vi "QCA - DUT Generate Tx Command.vi"(10 "Freq Index":i32, 11 "Standard Index":i32) -> (3 "Command Sent":string)   [LabVIEW 2011]
uses:
  niWLAN/WLAN -  niWLAN - INC - Select Measurement.ctl
panel:
  out "size(s)":i32
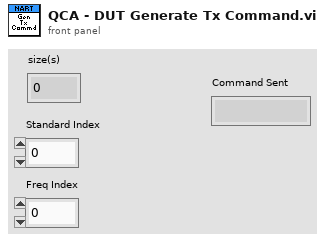
[diagram p1: front panel]
types:
  T1 = typedef "WLAN -  niWLAN - INC - Select Measurement.ctl" = cluster{"Tx_ 802.11a/g OFDM":bool, "Tx_ 802.11b DSSS/CCK":bool, "Tx_ 802.11n OFDM ":bool, "Tx_ 802.11ac OFDM ":bool}
  T2 = typedef "WLAN - TV - RW - INC - TV_DataType_Cluster.ctl" = cluster{"Standard":i32, "Channel Frequency(Hz)":dbl, "Power Level(dBm)":dbl, "Channel Bandwidth (Hz)":dbl, "Idle Interval(s)":dbl, "OFDM Data Rate (Mbps)":i32, "OFDM Payload Length (bytes)":i32, "Number of Packets":i32, "MCS Index":i32, "Guard Interval (s)":dbl, "80211n PLCP Frame Format":i32, "FEC Coding Type":i32, "DSSS Data Rate (Mbps)":i32, "DSSS Payload Length (bytes)":i32, "N_SS":i32}
  T3 = typedef "WLAN - TV - RW - INC - Tx_Measurement_Cluster.ctl" = cluster{"OFDM Advanced Controls(11ag)":T4, "DSSS Demod Parameters":T5, "OFDM Advanced Controls (11n)":T4, "OFDM Advanced Controls(11ac)":cluster{"OFDM Auto Compute Acquisition Length Enabled":i32, "OFDM Maximum Symbols Used":i32, "OFDM Time Tracking Enabled":i32, "OFDM Channel Tracking Enabled":i32, "OFDM Amplitude Tracking Enabled":i32, "OFDM CFO Estimation Method":i32, "OFDM Phase Tracking Method":i32, "OFDM Header Detection Enabled":i32, "OFDM MAC FCS Check Enabled":i32, "#Avg":i32, "#Iterations":i32}}
  T4 = typedef "WLAN - TV - RW - INC - TV_OFDM Demod.ctl" = cluster{"OFDM Auto Compute Acquisition Length Enabled":i32, "OFDM Maximum Symbols Used":i32, "OFDM Time Tracking Enabled":i32, "OFDM Channel Tracking Enabled":i32, "OFDM Amplitude Tracking Enabled":i32, "OFDM CFO Estimation Method":i32, "OFDM Phase Tracking Method":i32, "OFDM Header Detection Enabled":i32, "OFDM MAC FCS Check Enabled":i32, "#Avg":i32, "#Iterations":i32}
  T5 = typedef "WLAN - TV - RW - INC - TV_DSSS Demod.ctl" = cluster{"DSSS Auto Compute Acquisition Length Enabled":i32, "DSSS Equalization Enabled":i32, "DSSS Header Detection Enabled":i32, "DSSS MAC FCS Check Enabled":i32, "DSSS Measurement Start Location":i32, "DSSS Phase Tracking Method":i32, "DSSS Maximum Chips Used":i32, "DSSS Reference Pulse Shaping Filter":i32, "DSSS Reference Pulse Shaping Filter Coefficient":dbl, "# Avg":i32, "# Iterations":i32, "DSSS Power Ramp Enabled":i32}
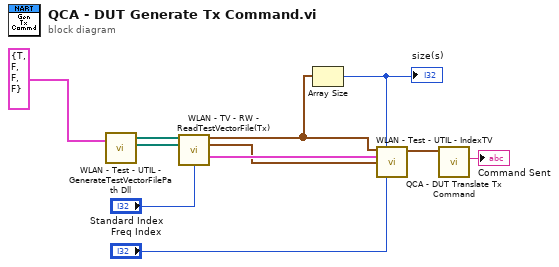
[diagram p0: block diagram]
diagram:
  n1 = call "WLAN - Test - UTIL - GenerateTestVectorFilePath Dll.vi"("Select Measurement"=T1 {"Tx_ 802.11a/g OFDM"=TRUE, "Tx_ 802.11b DSSS/CCK"=FALSE, "Tx_ 802.11n OFDM "=FALSE, "Tx_ 802.11ac OFDM "=FALSE} ("Select Standard")) -> ("TV Test Seq"=w10:path[], "TV Meas Config"=w9:path[])  [unwired: 11 in, 2 out]
  n2 = call "WLAN - TV - RW - ReadTestVectorFile(Tx).vi"("TX_TV_Sequence"=w10, "Measurment Settings"=w9, "Index"="Standard Index") -> ("TV's"=w6:T2[], "Tv First Element"=w7:T2, "WLAN Measurement Settings"=w8:T3)  [unwired: 8 in, 2 out]
  n3 = Array Size(array=w6) -> (size(s)=w5:i32)
  "size(s)" <- w5
  n4 = call "WLAN - Test - UTIL - IndexTV.vi"("TV"=w6, "N"=w5, "WLAN Measurement Settings"=w8, "Tv First Element"=w7, "Index"="Freq Index") -> ("TV"=w2:T2)  [unwired: 8 in, 2 out]
  n5 = call "QCA - DUT Translate Tx Command.vi"("TV Parameters(DataType)"=w2) -> ("Command Sent"=→"Command Sent":string)  [unwired: 8 in, 2 out]
